vi "MoveArm.vi"(8 "BackwardValue":dbl=-0.10000000000000014 min=-1.0 max=0.0 step=0.1, 9 "ForwardValue":dbl=0.10000000000000014 min=0.0 max=1.0 step=0.1, 10 "Direction":bool, 11 "Move Or Not":bool) -> (3 "Output":dbl)   [LabVIEW 2013]
doc: "moves the motor forwards or backwards depending on the state of the diretion boolean(true = forwards, false = backwards) input, and will move or turn off the motor according to the move or not boolean input."
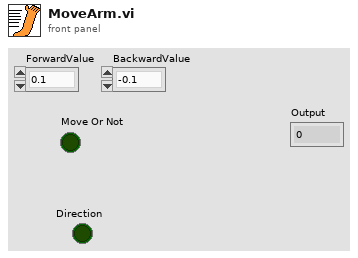
[diagram p1: front panel]
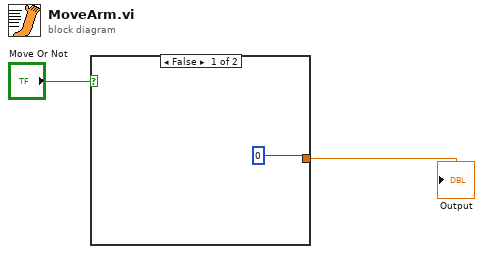
[diagram p0: block diagram]
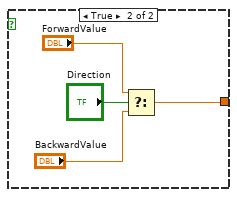
[diagram p2: hidden frame]
diagram:
  n1 = case shown="False" "Move Or Not" {
    tunnel: [0 w4] -> w1
    frame False {
    }
    frame True {
      n2 = Select(t="ForwardValue", s="Direction", f="BackwardValue") -> (s? t:f=w4:dbl)
    }
  }
  "Output" <- w1
